vi "Launch POLARIS TA Focus.vi"() -> ()   [LabVIEW 2014]
uses:
  <vilib>/userdefined/High Color/IMAQdx.ctl
  Utility/Width Method.ctl
  POLARIS Target Focus Actor/POLARIS Target Focus Actor.lvclass
  POLARIS Target Focus Actor/POLARIS Target Focus Actor.lvclass/POLARIS Target Focus Actor.ctl
  POLARIS Target Focus Actor/Write Method.vi
  Applications/HIJ Vision Camera App/HIJ Vision Camera App/Write Start Camera.vi
  Applications/HIJ Vision Camera App/HIJ Vision Camera App/Write my ConfigDir.vi
  Applications/HIJ Vision Camera App/HIJ Vision Camera App/Write my WorkDir.vi
  <vilib>/ActorFramework/Actor/Actor.lvclass
  Utility/POLARIS Vision utility.lvlib
panel:
  in  "Method":T1
  in  "Start WorkDir":path
  in  "Start ConfigDir":path
  in  "Start Camera":T2
  out "error out":errorcluster
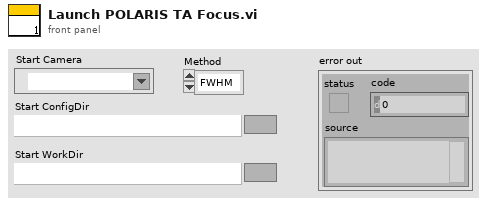
[diagram p1: front panel]
types:
  T1 = typedef "POLARIS Vision utility.lvlib/Width Method.ctl" = enum16{"FWHM", "1/e", "1/e^2", "80%", "90%"}
  T2 = typedef "IMAQdx.ctl" = refnum<k21>
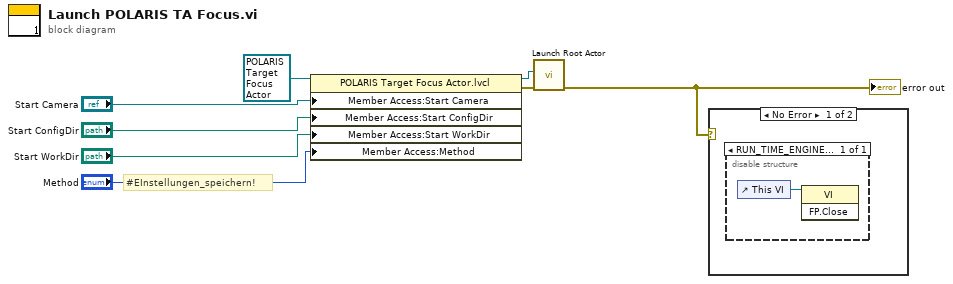
[diagram p0: block diagram]
diagram:
  # "#EInstellungen_speichern!"
  n1 = property class="POLARIS Target Focus Actor.lvcl"(reference=refnum<class "POLARIS Target Focus Actor.lvclass"> refnum ("POLARIS Target Focus Actor.lvlib:POLARIS Target Focus Actor.lvclass"), "Member Access:Start Camera"="Start Camera", "Member Access:Start ConfigDir"="Start ConfigDir", "Member Access:Start WorkDir"="Start WorkDir", "Member Access:Method"="Method") -> (reference out=w6:refnum<class "POLARIS Target Focus Actor.lvclass">, error out=w1:errorcluster)  [unwired: 1 in]
  n2 = call <vilib>:"Launch Root Actor.vi"("error in (no error)"=w1, "Actor"=w6) -> ("error out"=w7:errorcluster)  [unwired: 8 in, 1 out]
  "error out" <- w7
  n3 = case shown="No Error" w7 {
    frame No Error {
      n4 = disable-structure shown="RUN_TIME_ENGINE==True, Default" {
        frame condition #0 (active) {
          n5 = control-ref of="This VI"() -> (w9:refnum<vi>)
          n6 = invoke class="VI" method="FP.Close"(reference=w9) -> ()  [unwired: 2 in, 3 out]
        }
      }
    }
    frame Error {
    }
  }
